vi "Get Port Properties.vi"(8 "error in":errorcluster, 11 "port ref in":T1 format="%.0x") -> (0 "error out":errorcluster, 2 "channel configuration":T4, 3 "port ref out":T1 format="%.0x", 4 "found?":bool)   [LabVIEW 2020, in "AIM ARINC 429 Scripting.lvlib"]
uses:
  AIM ARINC 429 Scripting.lvlib
  Shared/Transfer Speed.ctl
  Shared/Direction.ctl
  <vilib>/NI VeriStand/Custom Device API/Custom Device Item Ref.ctl
  <vilib>/NI VeriStand/Custom Device API/Custom Device API.lvlib
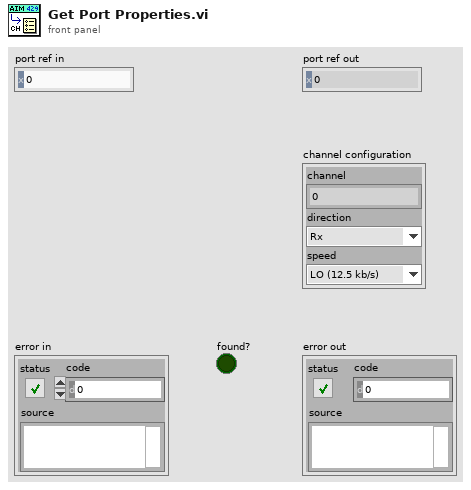
[diagram p1: front panel]
types:
  T1 = typedef "Custom Device API.lvlib/Custom Device Item Ref.ctl" = u64
  T2 = typedef "Direction.ctl" = enum16{"Rx", "Tx"}
  T3 = typedef "Transfer Speed.ctl" = enum16{"LO (12.5 kb/s)", "HI (100 kb/s)"}
  T4 = cluster{"channel":u8, "direction":T2, "speed":T3}
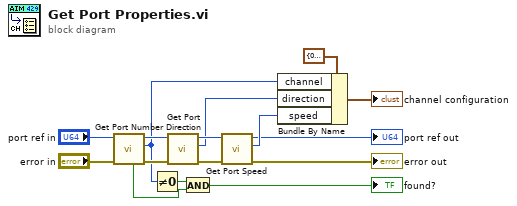
[diagram p0: block diagram]
diagram:
  n1 = call "Get Port Number.vi"("error in"="error in", "port ref in"="port ref in") -> ("error out"=w11:errorcluster, "port number"=w4:u16, "port ref out"=w8:T1, "found?"=w2:bool)  [unwired: 6 in]
  n2 = Not Equal To 0?(x=w4) -> (x != 0?=w3:bool)
  n3 = call "Get Port Direction.vi"("error in"=w11, "port ref in"=w8) -> ("error out"=w12:errorcluster, "direction"=w9:T2, "port ref out"=w13:T1)  [unwired: 7 in]
  n4 = And(x=w3, y=w2) -> (x .and. y?=→"found?":bool)
  n5 = call "Get Port Speed.vi"("error in"=w12, "port ref in"=w13) -> ("error out"=→"error out":errorcluster, "speed"=w15:T3, "port ref out"=→"port ref out":T1)  [unwired: 7 in]
  n6 = Bundle By Name(cluster=T4 {"channel"=0, "direction"=enum."Rx", "speed"=enum."LO (12.5 kb/s)"} ("active channel configuration"), "channel"=w4, "direction"=w9, "speed"=w15) -> (→"channel configuration":T4)
